vi "Results Packer.vi"(6 "PER":dbl, 7 "Command (Add)":T1, 8 "Test Frequency":u32, 9 "Test Paramaters":T2={"Interference sig. freq."=30, "Wanted Signal"=-67.0, "Blocking Signal"=-67.0, "Measurement res."=10} {"Measurement res." format="%.0f MHz"; "Blocking Signal" format="%#_gdBm"; "Interference sig. freq." format="%.0f MHz"; "Wanted Signal" format="%#_gdBm"}, 10 "Results":string, 11 "received Packets":u32) -> (1 "Pass":bool, 2 "Test Result Cluster":T3={"Test Frequency"=12750, "Received Packets"=0, "Results"="", "Test Paramaters"={"Interference sig. freq."=30, "Wanted Signal"=-67.0, "Blocking Signal"=-67.0, "Measurement res."=10}} {"Test Paramaters"."Measurement res." format="%.0f MHz"; "Test Paramaters"."Blocking Signal" format="%#_gdBm"; "Test Paramaters"."Interference sig. freq." format="%.0f MHz"; "Test Paramaters"."Wanted Signal" format="%#_gdBm"; "Test Frequency" format="%.0f MHz"}, 3 "Test Result Display Cluster":T4={"Test Frequency"=12750, "Percentage Error Rates"=0.0, "Results"=""} {"Percentage Error Rates" format="%.1f%%"; "Test Frequency" format="%.0f MHz"})   [LabVIEW 2013]
doc: "This VI will compile the results"
uses:
  Test Results Display Cluster.ctl
  Test Results Cluster.ctl
  Test Parameters.ctl
  Results FGV Command.ctl
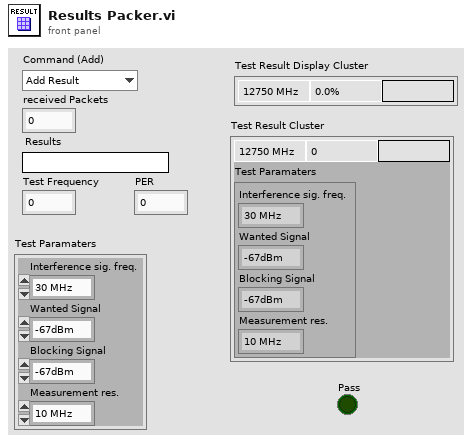
[diagram p1: front panel]
types:
  T1 = typedef "Results FGV Command.ctl" = enum16{"Add Result", "Return All", "Return fbf_1", "Return fbf_2", "Replace", "Clear All"}
  T2 = typedef "Test Parameters.ctl" = cluster{"Interference sig. freq.":u32, "Wanted Signal":dbl, "Blocking Signal":dbl, "Measurement res.":u32}
  T3 = typedef "Test Results Cluster.ctl" = cluster{"Test Frequency":u32, "Received Packets":u32, "Results":string, "Test Paramaters":T2}
  T4 = typedef "Test Results Display Cluster.ctl" = cluster{"Test Frequency":u32, "Percentage Error Rates":dbl, "Results":string}
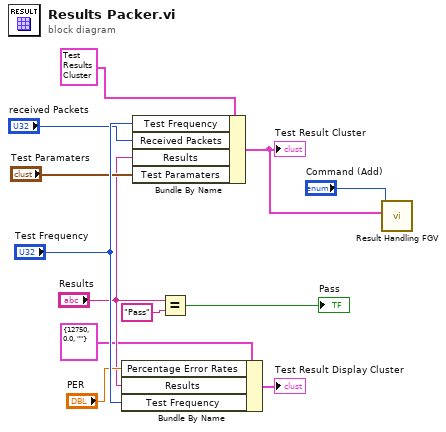
[diagram p0: block diagram]
diagram:
  n1 = Bundle By Name(cluster=T4 {"Test Frequency"=12750, "Percentage Error Rates"=0.0, "Results"=""} ("Test Result Display Cluster"), "Percentage Error Rates"="PER", "Results"="Results", "Test Frequency"="Test Frequency") -> (→"Test Result Display Cluster":T4)
  n2 = Bundle By Name(cluster=T3 {"Test Frequency"=12750, "Received Packets"=0, "Results"="", "Test Paramaters"={"Interference sig. freq."=30, "Wanted Signal"=-67.0, "Blocking Signal"=-67.0, "Measurement res."=10}} ("Test Result Cluster"), "Test Frequency"="Test Frequency", "Received Packets"="received Packets", "Results"="Results", "Test Paramaters"="Test Paramaters") -> (w6:T3)
  "Test Result Cluster" <- w6
  n3 = Equal?(x="Results", y="Pass") -> (x = y?=→"Pass":bool)
  n4 = call "Result Handling FGV.vi"("Test Result In"=w6, "Command"="Command (Add)") -> ()  [unwired: 8 in, 2 out]
